vi "LaserOnOffButtons.vi"() -> ()   [LabVIEW 2016]
panel:
  in  "ON/OFF":bool
  out "LASER":bool
  # "OFF"
  # "ON"
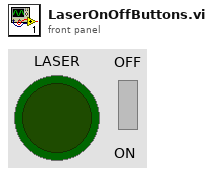
[diagram p1: front panel]
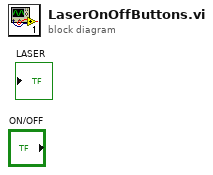
[diagram p0: block diagram]
diagram:
